vi "SelectsSRs(Poly).vi"   [LabVIEW 2018, in "DS_Lib.lvlib" / "SRReportParser.lvlib"]
uses:
  SRReportParser.lvlib
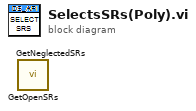
[diagram p0: block diagram]
diagram:
  n1 = call "GetOpenSRs.vi"() -> ()  [unwired: 8 in, 2 out]
  n2 = call "GetNeglectedSRs.vi"() -> ()  [unwired: 8 in, 2 out]
